vi "GetDeviceProperties.vi"(11 "device":T1) -> (2 "tdms properties":T9[](array[typedef]))   [LabVIEW 2017, in "Tdms.lvlib"]
doc: "Gets names and values of device-model properties that NI InsightCM Server requires TDMS files to contain. This VI also gets user-defined, or custom properties set in Systems Manager on the Device Configuration page>>Properties tab."
uses:
  <vilib>/addons/InsightCM/Utilities/Tdms/Tdms.lvlib
  <vilib>/addons/InsightCM/Utilities/Tdms/controls/Property.ctl
  <vilib>/addons/InsightCM/MessageBus/Base/controls/R2_Device.ctl
  <vilib>/addons/InsightCM/MessageBus/Base/controls/KeyValuePair.ctl
  <vilib>/addons/InsightCM/MessageBus/Base/controls/DeviceState.ctl
  <vilib>/addons/InsightCM/MessageBus/Base/controls/R2_DataGroup.ctl
  <vilib>/addons/InsightCM/MessageBus/Base/controls/OperatingState.ctl
  <vilib>/addons/InsightCM/MessageBus/Base/controls/Trigger.ctl
  <vilib>/addons/InsightCM/MessageBus/Base/controls/Condition.ctl
  <vilib>/addons/InsightCM/MessageBus/Base/controls/BurstModeTrigger.ctl
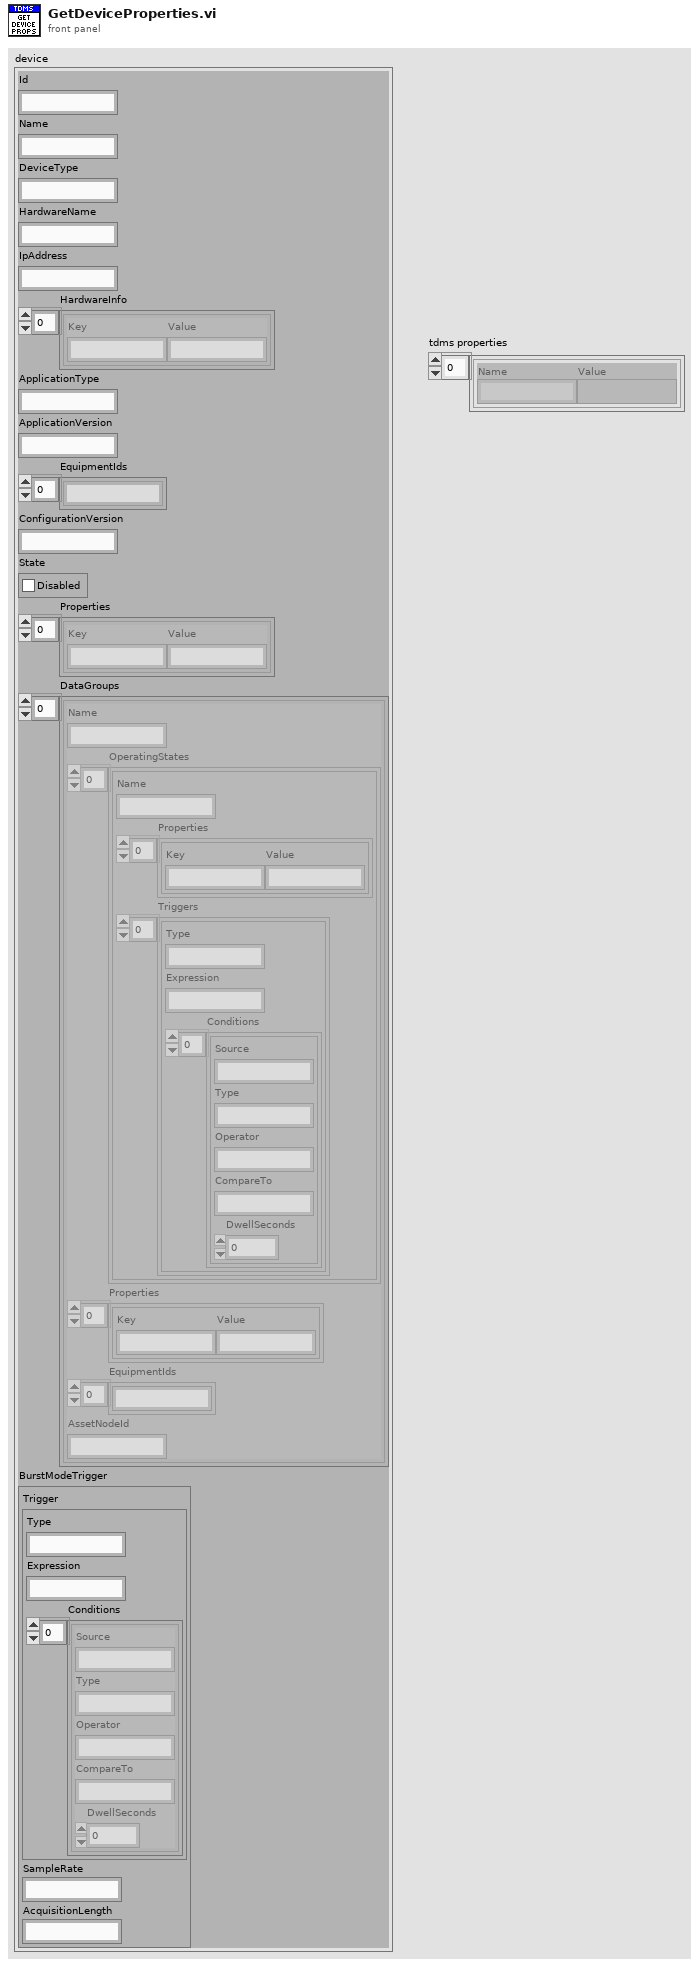
[diagram p1: front panel]
types:
  T1 = typedef "R2_Device.ctl" = cluster{"Id":string, "Name":string, "DeviceType":string, "HardwareName":string, "IpAddress":string, "HardwareInfo":T2[], "ApplicationType":string, "ApplicationVersion":string, "EquipmentIds":string[], "ConfigurationVersion":string, "State":T3, "Properties":T2[], "DataGroups":T4[], "BurstModeTrigger":T8}
  T2 = typedef "KeyValuePair.ctl" = cluster{"Key":string, "Value":string}
  T3 = typedef "DeviceState.ctl" = cluster{"Disabled":bool}
  T4 = typedef "R2_DataGroup.ctl" = cluster{"Name":string, "OperatingStates":T5[], "Properties":T2[], "EquipmentIds":string[], "AssetNodeId":string}
  T5 = typedef "OperatingState.ctl" = cluster{"Name":string, "Properties":T2[], "Triggers":T6[]}
  T6 = typedef "Trigger.ctl" = cluster{"Type":string, "Expression":string, "Conditions":T7[]}
  T7 = typedef "Condition.ctl" = cluster{"Source":string, "Type":string, "Operator":string, "CompareTo":string, "DwellSeconds":dbl}
  T8 = typedef "BurstModeTrigger.ctl" = cluster{"Trigger":T6, "SampleRate":string, "AcquisitionLength":string}
  T9 = typedef "Tdms.lvlib/Property.ctl" = cluster{"Name":string, "Value":variant}
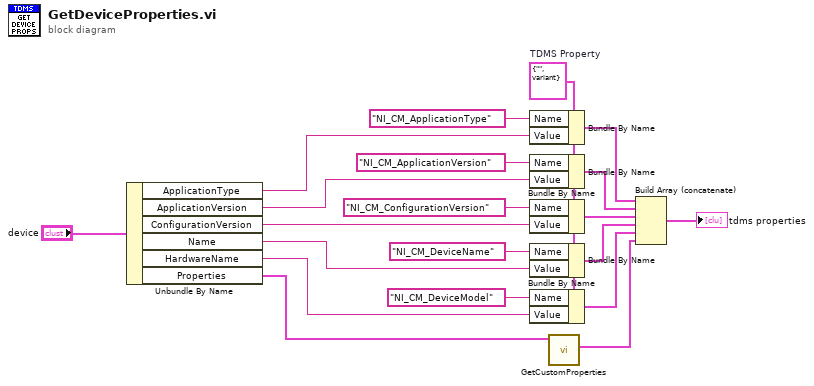
[diagram p0: block diagram]
diagram:
  w5 = T9 {"Name"="", "Value"=variant}  # TDMS Property
  n1 = Unbundle By Name("device") -> ("ApplicationType"=w1:string, "ApplicationVersion"=w2:string, "ConfigurationVersion"=w19:string, "Name"=w17:string, "HardwareName"=w11:string, "Properties"=w14:T2[])
  n2 = Bundle By Name(cluster=w5, "Name"="NI_CM_ApplicationType", "Value"=w1) -> (w3:T9)
  n3 = Bundle By Name(cluster=w5, "Name"="NI_CM_ApplicationVersion", "Value"=w2) -> (w4:T9)
  n4 = Bundle By Name(cluster=w5, "Name"="NI_CM_ConfigurationVersion", "Value"=w19) -> (w7:T9)
  n5 = Bundle By Name(cluster=w5, "Name"="NI_CM_DeviceName", "Value"=w17) -> (w12:T9)
  n6 = Bundle By Name(cluster=w5, "Name"="NI_CM_DeviceModel", "Value"=w11) -> (w9:T9)
  n7 = call <vilib>:"GetCustomProperties.vi"("Properties"=w14) -> ("Tdms Properties"=w10:T9[])  [unwired: 10 in]
  n8 = Build Array (concatenate)(w3, w4, w7, w12, w9, w10) -> (→"tdms properties":T9[])
